vi "输入数据解析.vi"(0 "单个参数补充":dbl, 1 "从板号":dbl=1.0, 2 "主板二维码":string="BNET01", 3 "从板二维码":string="BNET01", 5 "主板引用":refnum<vi>, 7 "从板引用":refnum<vi>, 9 "主板选项":string="三级故障阀值", 11 "枚举":enum16{"主板", "从板"}(ring), 12 "快换":bool caption="快换写入") -> (4 "输出数组":dbl[][](array[numeric]), 6 "数组长度":dbl[](array[numeric]), 8 "循环次数":i32, 10 "命令":u32, 14 "名称":string[](array[string]), 15 "命令序号":u32[](array[numeric]))   [LabVIEW 2013] (continued)
                # "极柱温度过高"
                n3831 = disable-structure shown="启用" {
                  disable-tunnel: w9952 -> [w9958 _]
                  disable-tunnel: [w9954 255 ("高字节1")] -> w9950
                  frame Disabled {
                    n3832 = Unbundle By Name(w9958) -> ("极柱温度过高"=w9957:dbl)
                    n3833 = call "输入分辨率计算-EV05.vi"("1字节?"=TRUE, "数值"=w9957, "偏移量"=-40.0, "分辨率"=1.0) -> ("高字节1"=w9954:dbl)  [unwired: 1 in, 6 out]
                  }
                  frame Enabled {
                  }
                }
                n3834 = Build Array(w9950) -> (w9951:i32[])
              }
              frame 16 {
                # "SOH过低"
                n3835 = disable-structure shown="启用" {
                  disable-tunnel: [w9975 w9983] -> w9962
                  disable-tunnel: w9961 -> [w9972 _]
                  disable-tunnel: [w9964 w9983] -> w9960
                  frame Disabled {
                    n3836 = Unbundle By Name(w9972) -> ("SOH过低"=w9971:dbl)
                    n3837 = call "输入分辨率计算-EV05.vi"("1字节?"=FALSE, "数值"=w9971, "偏移量"=0.0, "分辨率"=0.1) -> ("低字节"=w9973:dbl, "高字节1"=w9974:dbl)  [unwired: 1 in, 5 out]
                    n3838 = call "二进制解析-8.6.vi"("索引"=4, "数值"=w9974) -> ("低位子数组"=w9977:i32[])  [unwired: 3 out]
                    n3839 = call "二进制解析-8.6.vi"("索引"=4, "数值"=w9973) -> ("低位子数组"=w9966:i32[], "高位子数组"=w9976:i32[])  [unwired: 2 out]
                    n3840 = call "二进制解析-8.6.vi"("索引"=4, "数值"=0) -> ("低位子数组"=w9967:i32[])  [unwired: 3 out]
                    n3841 = Insert Into Array(array=w9977, new element=w9976) -> (w9970:i32[])  [unwired: 1 in]
                    n3842 = Insert Into Array(array=w9966, new element=w9967) -> (w9965:i32[])  [unwired: 1 in]
                    n3843 = call "数值二进制转十进制-8.6.vi"("子数组"=w9970) -> ("十进制数值"=w9975:i32)  [unwired: 4 out]
                    n3844 = call "数值二进制转十进制-8.6.vi"("子数组"=w9965) -> ("十进制数值"=w9964:i32)  [unwired: 4 out]
                  }
                  frame Enabled {
                    w9983 = 255 ("高字节1")
                  }
                }
                n3845 = Build Array(w9962, w9960) -> (w9963:i32[])
              }
            }
            n3846 = Insert Into Array(array=w9768, new element=w9769) -> (w9767:dbl[])  [unwired: 1 in]
          }
          n3847 = Build Array(w9764) -> (w9763:dbl[][])
          n3848 = Build Array("三级故障阀值") -> (w9754:string[])
        }
        frame "极柱温度过高" {
          n3849 = Unbundle By Name(w9989) -> ("一级故障"=w9990:refnum<vi>)
          n3850 = property class="Clust (严格)"(reference=w9990) -> ("Value"=w9988:T4)  [unwired: 1 in, 2 out]
          n3851 = for {
            N: 17 -> [_]
            tunnel: w9988 -> [w10000]
            shift-right: [w9997] -> w9994
            shift-left: dbl[] [] -> [w9998]
            i -> [w10001]
            n3852 = case shown="13" w10001 {
              tunnel: w10000 -> [w10002 w10013 w10024 w10034 w10044 w10054 w10066 w10078 w10090 w10102 w10114 w10126 w10140 w10161 w10173 w10182 w10191]
              tunnel: [w10003 w10014 w10025 w10035 w10045 w10056 w10068 w10080 w10092 w10104 w10116 w10127 w10149 w10164 w10172 w10181 w10193] -> w9999
              frame 0, Default {
                # "总电压过高"
                n3853 = disable-structure shown="启用" {
                  disable-tunnel: [w10009 w10012] -> w10005
                  disable-tunnel: [w10008 w10012] -> w10004
                  disable-tunnel: w10002 -> [w10007 _]
                  frame Disabled {
                    n3854 = Unbundle By Name(w10007) -> ("总电压过高"=w10006:dbl)
                    n3855 = call "输入分辨率计算-EV05.vi"("1字节?"=FALSE, "数值"=w10006, "分辨率"=0.1) -> ("低字节"=w10009:dbl, "高字节1"=w10008:dbl)  [unwired: 2 in, 5 out]
                  }
                  frame Enabled {
                    w10012 = 255 ("高字节1")
                  }
                }
                n3856 = Build Array(w10004, w10005) -> (w10003:i32[])
              }
              frame 1 {
                # "总电压过低"
                n3857 = disable-structure shown="启用" {
                  disable-tunnel: [w10020 w10023] -> w10016
                  disable-tunnel: [w10019 w10023] -> w10015
                  disable-tunnel: w10013 -> [w10018 _]
                  frame Disabled {
                    n3858 = Unbundle By Name(w10018) -> ("总电压过低"=w10017:dbl)
                    n3859 = call "输入分辨率计算-EV05.vi"("1字节?"=FALSE, "数值"=w10017, "分辨率"=0.1) -> ("低字节"=w10020:dbl, "高字节1"=w10019:dbl)  [unwired: 2 in, 5 out]
                  }
                  frame Enabled {
                    w10023 = 255 ("高字节1")
                  }
                }
                n3860 = Build Array(w10015, w10016) -> (w10014:i32[])
              }
              frame 2 {
                # "温度过高"
                n3861 = disable-structure shown="启用" {
                  disable-tunnel: [w10030 255 ("高字节1")] -> w10026
                  disable-tunnel: w10024 -> [w10028 _]
                  frame Disabled {
                    n3862 = Unbundle By Name(w10028) -> ("温度过高"=w10027:dbl)
                    n3863 = call "输入分辨率计算-EV05.vi"("1字节?"=TRUE, "数值"=w10027, "偏移量"=-40.0, "分辨率"=1.0) -> ("高字节1"=w10030:dbl)  [unwired: 1 in, 6 out]
                  }
                  frame Enabled {
                  }
                }
                n3864 = Build Array(w10026) -> (w10025:i32[])
              }
              frame 3 {
                # "温度过低"
                n3865 = disable-structure shown="启用" {
                  disable-tunnel: [w10040 255 ("高字节1")] -> w10036
                  disable-tunnel: w10034 -> [w10038 _]
                  frame Disabled {
                    n3866 = Unbundle By Name(w10038) -> ("温度过低"=w10037:dbl)
                    n3867 = call "输入分辨率计算-EV05.vi"("1字节?"=TRUE, "数值"=w10037, "偏移量"=-40.0, "分辨率"=1.0) -> ("高字节1"=w10040:dbl)  [unwired: 1 in, 6 out]
                  }
                  frame Enabled {
                  }
                }
                n3868 = Build Array(w10036) -> (w10035:i32[])
              }
              frame 4 {
                # "整组温度不均衡"
                n3869 = disable-structure shown="启用" {
                  disable-tunnel: [w10050 255 ("高字节1")] -> w10046
                  disable-tunnel: w10044 -> [w10048 _]
                  frame Disabled {
                    n3870 = Unbundle By Name(w10048) -> ("整组温度不均衡"=w10047:dbl)
                    n3871 = call "输入分辨率计算-EV05.vi"("1字节?"=TRUE, "数值"=w10047, "偏移量"=0.0, "分辨率"=1.0) -> ("高字节1"=w10050:dbl)  [unwired: 1 in, 6 out]
                  }
                  frame Enabled {
                  }
                }
                n3872 = Build Array(w10046) -> (w10045:i32[])
              }
              frame 5 {
                # "单组电压不均衡"
                n3873 = disable-structure shown="启用" {
                  disable-tunnel: [w10062 w10065] -> w10057
                  disable-tunnel: [w10060 w10065] -> w10055
                  disable-tunnel: w10054 -> [w10059 _]
                  frame Disabled {
                    n3874 = Unbundle By Name(w10059) -> ("单组电压不均衡"=w10058:dbl)
                    n3875 = call "输入分辨率计算-EV05.vi"("1字节?"=FALSE, "数值"=w10058, "偏移量"=0.0, "分辨率"=0.001) -> ("低字节"=w10060:dbl, "高字节1"=w10062:dbl)  [unwired: 1 in, 5 out]
                  }
                  frame Enabled {
                    w10065 = 255 ("高字节1")
                  }
                }
                n3876 = Build Array(w10057, w10055) -> (w10056:i32[])
              }
              frame 6 {
                # "整组电压不均衡"
                n3877 = disable-structure shown="启用" {
                  disable-tunnel: [w10074 w10077] -> w10069
                  disable-tunnel: [w10072 w10077] -> w10067
                  disable-tunnel: w10066 -> [w10071 _]
                  frame Disabled {
                    n3878 = Unbundle By Name(w10071) -> ("整组电压不均衡"=w10070:dbl)
                    n3879 = call "输入分辨率计算-EV05.vi"("1字节?"=FALSE, "数值"=w10070, "偏移量"=0.0, "分辨率"=0.001) -> ("低字节"=w10072:dbl, "高字节1"=w10074:dbl)  [unwired: 1 in, 5 out]
                  }
                  frame Enabled {
                    w10077 = 255 ("高字节1")
                  }
                }
                n3880 = Build Array(w10069, w10067) -> (w10068:i32[])
              }
              frame 7 {
                # "单体电压过高"
                n3881 = disable-structure shown="启用" {
                  disable-tunnel: [w10086 w10089] -> w10081
                  disable-tunnel: [w10084 w10089] -> w10079
                  disable-tunnel: w10078 -> [w10083 _]
                  frame Disabled {
                    n3882 = Unbundle By Name(w10083) -> ("单体电压过高"=w10082:dbl)
                    n3883 = call "输入分辨率计算-EV05.vi"("1字节?"=FALSE, "数值"=w10082, "偏移量"=0.0, "分辨率"=0.001) -> ("低字节"=w10084:dbl, "高字节1"=w10086:dbl)  [unwired: 1 in, 5 out]
                  }
                  frame Enabled {
                    w10089 = 255 ("高字节1")
                  }
                }
                n3884 = Build Array(w10081, w10079) -> (w10080:i32[])
              }
              frame 8 {
                # "单体电压过低"
                n3885 = disable-structure shown="启用" {
                  disable-tunnel: [w10098 w10101] -> w10093
                  disable-tunnel: [w10096 w10101] -> w10091
                  disable-tunnel: w10090 -> [w10095 _]
                  frame Disabled {
                    n3886 = Unbundle By Name(w10095) -> ("单体电压过低"=w10094:dbl)
                    n3887 = call "输入分辨率计算-EV05.vi"("1字节?"=FALSE, "数值"=w10094, "偏移量"=0.0, "分辨率"=0.001) -> ("低字节"=w10096:dbl, "高字节1"=w10098:dbl)  [unwired: 1 in, 5 out]
                  }
                  frame Enabled {
                    w10101 = 255 ("高字节1")
                  }
                }
                n3888 = Build Array(w10093, w10091) -> (w10092:i32[])
              }
              frame 9 {
                # "充电电流过高"
                n3889 = disable-structure shown="启用" {
                  disable-tunnel: [w10110 w10113] -> w10105
                  disable-tunnel: [w10108 w10113] -> w10103
                  disable-tunnel: w10102 -> [w10107 _]
                  frame Disabled {
                    n3890 = Unbundle By Name(w10107) -> ("充电电流过高"=w10106:dbl)
                    n3891 = call "输入分辨率计算-EV05.vi"("1字节?"=FALSE, "数值"=w10106, "偏移量"=-3000.0, "分辨率"=0.1) -> ("低字节"=w10108:dbl, "高字节1"=w10110:dbl)  [unwired: 1 in, 5 out]
                  }
                  frame Enabled {
                    w10113 = 255 ("高字节1")
                  }
                }
                n3892 = Build Array(w10105, w10103) -> (w10104:i32[])
              }
              frame 10 {
                # "放电电流过高"
                n3893 = disable-structure shown="启用" {
                  disable-tunnel: [w10122 w10125] -> w10117
                  disable-tunnel: [w10120 w10125] -> w10115
                  disable-tunnel: w10114 -> [w10119 _]
                  frame Disabled {
                    n3894 = Unbundle By Name(w10119) -> ("放电电流过高"=w10118:dbl)
                    n3895 = call "输入分辨率计算-EV05.vi"("1字节?"=FALSE, "数值"=w10118, "偏移量"=-3000.0, "分辨率"=0.1) -> ("低字节"=w10120:dbl, "高字节1"=w10122:dbl)  [unwired: 1 in, 5 out]
                  }
                  frame Enabled {
                    w10125 = 255 ("高字节1")
                  }
                }
                n3896 = Build Array(w10117, w10115) -> (w10116:i32[])
              }
              frame 11 {
                # "单组温度不均衡"
                n3897 = disable-structure shown="启用" {
                  disable-tunnel: [w10132 255 ("高字节1")] -> w10128
                  disable-tunnel: w10126 -> [w10130 _]
                  frame Disabled {
                    n3898 = Unbundle By Name(w10130) -> ("单组温度不均衡"=w10129:dbl)
                    n3899 = call "输入分辨率计算-EV05.vi"("1字节?"=TRUE, "数值"=w10129, "偏移量"=0.0, "分辨率"=1.0) -> ("高字节1"=w10132:dbl)  [unwired: 1 in, 6 out]
                  }
                  frame Enabled {
                  }
                }
                n3900 = Build Array(w10128) -> (w10127:i32[])
              }
              frame 12 {
                # "SOC过高"
                n3901 = Unbundle By Name(w10140) -> ("SOC过高"=w10139:dbl)
                n3902 = call "输入分辨率计算-EV05.vi"("1字节?"=FALSE, "数值"=w10139, "偏移量"=0.0, "分辨率"=0.1) -> ("低字节"=w10141:dbl, "高字节1"=w10142:dbl)  [unwired: 1 in, 5 out]
                n3903 = call "二进制解析-8.6.vi"("索引"=4, "数值"=w10142) -> ("低位子数组"=w10145:i32[])  [unwired: 3 out]
                n3904 = call "二进制解析-8.6.vi"("索引"=4, "数值"=w10141) -> ("低位子数组"=w10137:i32[], "高位子数组"=w10144:i32[])  [unwired: 2 out]
                n3905 = Insert Into Array(array=w10145, new element=w10144) -> (w10143:i32[])  [unwired: 1 in]
                n3906 = call "数值二进制转十进制-8.6.vi"("子数组"=w10143) -> ("十进制数值"=w10138:i32)  [unwired: 4 out]
                n3907 = disable-structure shown="启用" {
                  disable-tunnel: w10138 -> [w10153 _]
                  disable-tunnel: [w10153 255 ("高字节1")] -> w10136
                  disable-tunnel: w10137 -> [w10152 _]
                  disable-tunnel: [w10152 i32[] [] ("低位子数组 29")] -> _
                  frame Disabled {
                  }
                  frame Enabled {
                  }
                }
                n3908 = Build Array(w10136, w10136) -> (w10149:i32[])
              }
              frame 13 {
                # "SOC过低"
                n3909 = Unbundle By Name(w10161) -> ("SOC过低"=w10160:dbl)
                n3910 = call "输入分辨率计算-EV05.vi"("1字节?"=FALSE, "数值"=w10160, "偏移量"=0.0, "分辨率"=0.1) -> ("低字节"=w10158:dbl, "高字节1"=w10159:dbl)  [unwired: 1 in, 5 out]
                n3911 = call "二进制解析-8.6.vi"("索引"=4, "数值"=w10159) -> ("低位子数组"=w10157:i32[])  [unwired: 3 out]
                n3912 = disable-structure shown="启用" {
                  disable-tunnel: w10158 -> [w10168 _]
                  disable-tunnel: [w10168 255 ("高字节1")] -> w10156
                  disable-tunnel: w10157 -> [w10167 _]
                  disable-tunnel: [w10167 i32[] [] ("低位子数组")] -> _
                  frame Disabled {
                    (unwired) i32[] [] ("低位子数组 4")
                  }
                  frame Enabled {
                  }
                }
                n3913 = Build Array(w10156, w10156) -> (w10164:i32[])
              }
              frame 14 {
                # "内阻过大"
                n3914 = disable-structure shown="启用" {
                  disable-tunnel: w10173 -> [w10178 _]
                  disable-tunnel: [w10174 255 ("高字节1")] -> w10171
                  frame Disabled {
                    n3915 = Unbundle By Name(w10178) -> ("内阻过大"=w10177:dbl)
                    n3916 = call "输入分辨率计算-EV05.vi"("1字节?"=TRUE, "数值"=w10177, "分辨率"=0.1) -> ("高字节1"=w10174:dbl)  [unwired: 2 in, 6 out]
                  }
                  frame Enabled {
                  }
                }
                n3917 = Build Array(w10171) -> (w10172:i32[])
              }
              frame 15 {
                # "极柱温度过高"
                n3918 = disable-structure shown="启用" {
                  disable-tunnel: w10182 -> [w10188 _]
                  disable-tunnel: [w10184 255 ("高字节1")] -> w10180
                  frame Enabled {
                    n3919 = Unbundle By Name(w10188) -> ("极柱温度过高"=w10187:dbl)
                    n3920 = call "输入分辨率计算-EV05.vi"("1字节?"=TRUE, "数值"=w10187, "偏移量"=-40.0, "分辨率"=1.0) -> ("高字节1"=w10184:dbl)  [unwired: 1 in, 6 out]
                  }
                  frame Disabled {
                  }
                }
                n3921 = Build Array(w10180) -> (w10181:dbl[])
              }
              frame 16 {
                # "SOH过低"
                n3922 = disable-structure shown="启用" {
                  disable-tunnel: [w10205 w10213] -> w10192
                  disable-tunnel: w10191 -> [w10202 _]
                  disable-tunnel: [w10194 w10213] -> w10190
                  frame Disabled {
                    n3923 = Unbundle By Name(w10202) -> ("SOH过低"=w10201:dbl)
                    n3924 = call "输入分辨率计算-EV05.vi"("1字节?"=FALSE, "数值"=w10201, "偏移量"=0.0, "分辨率"=0.1) -> ("低字节"=w10203:dbl, "高字节1"=w10204:dbl)  [unwired: 1 in, 5 out]
                    n3925 = call "二进制解析-8.6.vi"("索引"=4, "数值"=w10204) -> ("低位子数组"=w10207:i32[])  [unwired: 3 out]
                    n3926 = call "二进制解析-8.6.vi"("索引"=4, "数值"=w10203) -> ("低位子数组"=w10196:i32[], "高位子数组"=w10206:i32[])  [unwired: 2 out]
                    n3927 = call "二进制解析-8.6.vi"("索引"=4, "数值"=0) -> ("低位子数组"=w10197:i32[])  [unwired: 3 out]
                    n3928 = Insert Into Array(array=w10207, new element=w10206) -> (w10200:i32[])  [unwired: 1 in]
                    n3929 = Insert Into Array(array=w10196, new element=w10197) -> (w10195:i32[])  [unwired: 1 in]
                    n3930 = call "数值二进制转十进制-8.6.vi"("子数组"=w10200) -> ("十进制数值"=w10205:i32)  [unwired: 4 out]
                    n3931 = call "数值二进制转十进制-8.6.vi"("子数组"=w10195) -> ("十进制数值"=w10194:i32)  [unwired: 4 out]
                  }
                  frame Enabled {
                    w10213 = 255 ("高字节1")
                  }
                }
                n3932 = Build Array(w10192, w10190) -> (w10193:i32[])
              }
            }
            n3933 = Insert Into Array(array=w9998, new element=w9999) -> (w9997:dbl[])  [unwired: 1 in]
          }
          n3934 = Build Array(w9994) -> (w9993:dbl[][])
          n3935 = Build Array("一级故障阀值") -> (w9984:string[])
        }
        frame "极柱温度过高(2)" {
          n3936 = Unbundle By Name(w10219) -> ("一级故障 2"=w10220:refnum<vi>)
          n3937 = property class="Clust (严格)"(reference=w10220) -> ("Value"=w10218:T4)  [unwired: 1 in, 2 out]
          n3938 = for {
            N: 17 -> [_]
            tunnel: w10218 -> [w10230]
            shift-right: [w10227] -> w10224
            shift-left: dbl[] [] -> [w10228]
            i -> [w10231]
            n3939 = case shown="13" w10231 {
              tunnel: w10230 -> [w10232 w10243 w10254 w10264 w10274 w10284 w10296 w10308 w10320 w10332 w10344 w10356 w10370 w10391 w10403 w10412 w10421]
              tunnel: [w10233 w10244 w10255 w10265 w10275 w10286 w10298 w10310 w10322 w10334 w10346 w10357 w10379 w10394 w10402 w10411 w10423] -> w10229
              frame 0, Default {
                # "总电压过高"
                n3940 = disable-structure shown="启用" {
                  disable-tunnel: [w10239 w10242] -> w10235
                  disable-tunnel: [w10238 w10242] -> w10234
                  disable-tunnel: w10232 -> [w10237 _]
                  frame Disabled {
                    n3941 = Unbundle By Name(w10237) -> ("总电压过高"=w10236:dbl)
                    n3942 = call "输入分辨率计算-EV05.vi"("1字节?"=FALSE, "数值"=w10236, "分辨率"=0.1) -> ("低字节"=w10239:dbl, "高字节1"=w10238:dbl)  [unwired: 2 in, 5 out]
                  }
                  frame Enabled {
                    w10242 = 255 ("高字节1")
                  }
                }
                n3943 = Build Array(w10234, w10235) -> (w10233:i32[])
              }
              frame 1 {
                # "总电压过低"
                n3944 = disable-structure shown="启用" {
                  disable-tunnel: [w10250 w10253] -> w10246
                  disable-tunnel: [w10249 w10253] -> w10245
                  disable-tunnel: w10243 -> [w10248 _]
                  frame Disabled {
                    n3945 = Unbundle By Name(w10248) -> ("总电压过低"=w10247:dbl)
                    n3946 = call "输入分辨率计算-EV05.vi"("1字节?"=FALSE, "数值"=w10247, "分辨率"=0.1) -> ("低字节"=w10250:dbl, "高字节1"=w10249:dbl)  [unwired: 2 in, 5 out]
                  }
                  frame Enabled {
                    w10253 = 255 ("高字节1")
                  }
                }
                n3947 = Build Array(w10245, w10246) -> (w10244:i32[])
              }
              frame 2 {
                # "温度过高"
                n3948 = disable-structure shown="启用" {
                  disable-tunnel: [w10260 255 ("高字节1")] -> w10256
                  disable-tunnel: w10254 -> [w10258 _]
                  frame Disabled {
                    n3949 = Unbundle By Name(w10258) -> ("温度过高"=w10257:dbl)
                    n3950 = call "输入分辨率计算-EV05.vi"("1字节?"=TRUE, "数值"=w10257, "偏移量"=-40.0, "分辨率"=1.0) -> ("高字节1"=w10260:dbl)  [unwired: 1 in, 6 out]
                  }
                  frame Enabled {
                  }
                }
                n3951 = Build Array(w10256) -> (w10255:i32[])
              }
              frame 3 {
                # "温度过低"
                n3952 = disable-structure shown="启用" {
                  disable-tunnel: [w10270 255 ("高字节1")] -> w10266
                  disable-tunnel: w10264 -> [w10268 _]
                  frame Disabled {
                    n3953 = Unbundle By Name(w10268) -> ("温度过低"=w10267:dbl)
                    n3954 = call "输入分辨率计算-EV05.vi"("1字节?"=TRUE, "数值"=w10267, "偏移量"=-40.0, "分辨率"=1.0) -> ("高字节1"=w10270:dbl)  [unwired: 1 in, 6 out]
                  }
                  frame Enabled {
                  }
                }
                n3955 = Build Array(w10266) -> (w10265:i32[])
              }
              frame 4 {
                # "整组温度不均衡"
                n3956 = disable-structure shown="启用" {
                  disable-tunnel: [w10280 255 ("高字节1")] -> w10276
                  disable-tunnel: w10274 -> [w10278 _]
                  frame Disabled {
                    n3957 = Unbundle By Name(w10278) -> ("整组温度不均衡"=w10277:dbl)
                    n3958 = call "输入分辨率计算-EV05.vi"("1字节?"=TRUE, "数值"=w10277, "偏移量"=0.0, "分辨率"=1.0) -> ("高字节1"=w10280:dbl)  [unwired: 1 in, 6 out]
                  }
                  frame Enabled {
                  }
                }
                n3959 = Build Array(w10276) -> (w10275:i32[])
              }
              frame 5 {
                # "单组电压不均衡"
                n3960 = disable-structure shown="启用" {
                  disable-tunnel: [w10292 w10295] -> w10287
                  disable-tunnel: [w10290 w10295] -> w10285
                  disable-tunnel: w10284 -> [w10289 _]
                  frame Disabled {
                    n3961 = Unbundle By Name(w10289) -> ("单组电压不均衡"=w10288:dbl)
                    n3962 = call "输入分辨率计算-EV05.vi"("1字节?"=FALSE, "数值"=w10288, "偏移量"=0.0, "分辨率"=0.001) -> ("低字节"=w10290:dbl, "高字节1"=w10292:dbl)  [unwired: 1 in, 5 out]
                  }
                  frame Enabled {
                    w10295 = 255 ("高字节1")
                  }
                }
                n3963 = Build Array(w10287, w10285) -> (w10286:i32[])
              }
              frame 6 {
                # "整组电压不均衡"
                n3964 = disable-structure shown="启用" {
                  disable-tunnel: [w10304 w10307] -> w10299
                  disable-tunnel: [w10302 w10307] -> w10297
                  disable-tunnel: w10296 -> [w10301 _]
                  frame Disabled {
                    n3965 = Unbundle By Name(w10301) -> ("整组电压不均衡"=w10300:dbl)
                    n3966 = call "输入分辨率计算-EV05.vi"("1字节?"=FALSE, "数值"=w10300, "偏移量"=0.0, "分辨率"=0.001) -> ("低字节"=w10302:dbl, "高字节1"=w10304:dbl)  [unwired: 1 in, 5 out]
                  }
                  frame Enabled {
                    w10307 = 255 ("高字节1")
                  }
                }
                n3967 = Build Array(w10299, w10297) -> (w10298:i32[])
              }
              frame 7 {
                # "单体电压过高"
                n3968 = disable-structure shown="启用" {
                  disable-tunnel: [w10316 w10319] -> w10311
                  disable-tunnel: [w10314 w10319] -> w10309
                  disable-tunnel: w10308 -> [w10313 _]
                  frame Disabled {
                    n3969 = Unbundle By Name(w10313) -> ("单体电压过高"=w10312:dbl)
                    n3970 = call "输入分辨率计算-EV05.vi"("1字节?"=FALSE, "数值"=w10312, "偏移量"=0.0, "分辨率"=0.001) -> ("低字节"=w10314:dbl, "高字节1"=w10316:dbl)  [unwired: 1 in, 5 out]
                  }
                  frame Enabled {
                    w10319 = 255 ("高字节1")
                  }
                }
                n3971 = Build Array(w10311, w10309) -> (w10310:i32[])
              }
              frame 8 {
                # "单体电压过低"
                n3972 = disable-structure shown="启用" {
                  disable-tunnel: [w10328 w10331] -> w10323
                  disable-tunnel: [w10326 w10331] -> w10321
                  disable-tunnel: w10320 -> [w10325 _]
                  frame Disabled {
                    n3973 = Unbundle By Name(w10325) -> ("单体电压过低"=w10324:dbl)
                    n3974 = call "输入分辨率计算-EV05.vi"("1字节?"=FALSE, "数值"=w10324, "偏移量"=0.0, "分辨率"=0.001) -> ("低字节"=w10326:dbl, "高字节1"=w10328:dbl)  [unwired: 1 in, 5 out]
                  }
                  frame Enabled {
                    w10331 = 255 ("高字节1")
                  }
                }
                n3975 = Build Array(w10323, w10321) -> (w10322:i32[])
              }
              frame 9 {
                # "充电电流过高"
                n3976 = disable-structure shown="启用" {
                  disable-tunnel: [w10340 w10343] -> w10335
                  disable-tunnel: [w10338 w10343] -> w10333
                  disable-tunnel: w10332 -> [w10337 _]
                  frame Disabled {
                    n3977 = Unbundle By Name(w10337) -> ("充电电流过高"=w10336:dbl)
                    n3978 = call "输入分辨率计算-EV05.vi"("1字节?"=FALSE, "数值"=w10336, "偏移量"=-3000.0, "分辨率"=0.1) -> ("低字节"=w10338:dbl, "高字节1"=w10340:dbl)  [unwired: 1 in, 5 out]
                  }
                  frame Enabled {
                    w10343 = 255 ("高字节1")
                  }
                }
                n3979 = Build Array(w10335, w10333) -> (w10334:i32[])
              }
              frame 10 {
                # "放电电流过高"
                n3980 = disable-structure shown="启用" {
                  disable-tunnel: [w10352 w10355] -> w10347
                  disable-tunnel: [w10350 w10355] -> w10345
                  disable-tunnel: w10344 -> [w10349 _]
                  frame Disabled {
                    n3981 = Unbundle By Name(w10349) -> ("放电电流过高"=w10348:dbl)
                    n3982 = call "输入分辨率计算-EV05.vi"("1字节?"=FALSE, "数值"=w10348, "偏移量"=-3000.0, "分辨率"=0.1) -> ("低字节"=w10350:dbl, "高字节1"=w10352:dbl)  [unwired: 1 in, 5 out]
                  }
                  frame Enabled {
                    w10355 = 255 ("高字节1")
                  }
                }
                n3983 = Build Array(w10347, w10345) -> (w10346:i32[])
              }
              frame 11 {
                # "单组温度不均衡"
                n3984 = disable-structure shown="启用" {
                  disable-tunnel: [w10362 255 ("高字节1")] -> w10358
                  disable-tunnel: w10356 -> [w10360 _]
                  frame Disabled {
                    n3985 = Unbundle By Name(w10360) -> ("单组温度不均衡"=w10359:dbl)
                    n3986 = call "输入分辨率计算-EV05.vi"("1字节?"=TRUE, "数值"=w10359, "偏移量"=0.0, "分辨率"=1.0) -> ("高字节1"=w10362:dbl)  [unwired: 1 in, 6 out]
                  }
                  frame Enabled {
                  }
                }
                n3987 = Build Array(w10358) -> (w10357:i32[])
              }
              frame 12 {
                # "SOC过高"
                n3988 = Unbundle By Name(w10370) -> ("SOC过高"=w10369:dbl)
                n3989 = call "输入分辨率计算-EV05.vi"("1字节?"=FALSE, "数值"=w10369, "偏移量"=0.0, "分辨率"=0.1) -> ("低字节"=w10371:dbl, "高字节1"=w10372:dbl)  [unwired: 1 in, 5 out]
                n3990 = call "二进制解析-8.6.vi"("索引"=4, "数值"=w10372) -> ("低位子数组"=w10375:i32[])  [unwired: 3 out]
                n3991 = call "二进制解析-8.6.vi"("索引"=4, "数值"=w10371) -> ("低位子数组"=w10367:i32[], "高位子数组"=w10374:i32[])  [unwired: 2 out]
                n3992 = Insert Into Array(array=w10375, new element=w10374) -> (w10373:i32[])  [unwired: 1 in]
                n3993 = call "数值二进制转十进制-8.6.vi"("子数组"=w10373) -> ("十进制数值"=w10368:i32)  [unwired: 4 out]
                n3994 = disable-structure shown="启用" {
                  disable-tunnel: w10368 -> [w10383 _]
                  disable-tunnel: [w10383 255 ("高字节1")] -> w10366
                  disable-tunnel: w10367 -> [w10382 _]
                  disable-tunnel: [w10382 i32[] [] ("低位子数组 29")] -> _
                  frame Disabled {
                  }
                  frame Enabled {
                  }
                }
                n3995 = Build Array(w10366, w10366) -> (w10379:i32[])
              }
              frame 13 {
                # "SOC过低"
                n3996 = Unbundle By Name(w10391) -> ("SOC过低"=w10390:dbl)
                n3997 = call "输入分辨率计算-EV05.vi"("1字节?"=FALSE, "数值"=w10390, "偏移量"=0.0, "分辨率"=0.1) -> ("低字节"=w10388:dbl, "高字节1"=w10389:dbl)  [unwired: 1 in, 5 out]
                n3998 = call "二进制解析-8.6.vi"("索引"=4, "数值"=w10389) -> ("低位子数组"=w10387:i32[])  [unwired: 3 out]
                n3999 = disable-structure shown="启用" {
                  disable-tunnel: w10388 -> [w10398 _]
                  disable-tunnel: [w10398 255 ("高字节1")] -> w10386
                  disable-tunnel: w10387 -> [w10397 _]
                  disable-tunnel: [w10397 i32[] [] ("低位子数组")] -> _
                  frame Disabled {
                    (unwired) i32[] [] ("低位子数组 4")
                  }
                  frame Enabled {
                  }
                }
                n4000 = Build Array(w10386, w10386) -> (w10394:i32[])
              }
              frame 14 {
                # "内阻过大"
                n4001 = disable-structure shown="启用" {
                  disable-tunnel: w10403 -> [w10408 _]
                  disable-tunnel: [w10404 255 ("高字节1")] -> w10401
                  frame Disabled {
                    n4002 = Unbundle By Name(w10408) -> ("内阻过大"=w10407:dbl)
                    n4003 = call "输入分辨率计算-EV05.vi"("1字节?"=TRUE, "数值"=w10407, "分辨率"=0.1) -> ("高字节1"=w10404:dbl)  [unwired: 2 in, 6 out]
                  }
                  frame Enabled {
                  }
                }
                n4004 = Build Array(w10401) -> (w10402:i32[])
              }
              frame 15 {
                # "极柱温度过高"
                n4005 = disable-structure shown="启用" {
                  disable-tunnel: w10412 -> [w10418 _]
                  disable-tunnel: [w10414 255 ("高字节1")] -> w10410
                  frame Enabled {
                    n4006 = Unbundle By Name(w10418) -> ("极柱温度过高"=w10417:dbl)
                    n4007 = call "输入分辨率计算-EV05.vi"("1字节?"=TRUE, "数值"=w10417, "偏移量"=-40.0, "分辨率"=1.0) -> ("高字节1"=w10414:dbl)  [unwired: 1 in, 6 out]
                  }
                  frame Disabled {
                  }
                }
                n4008 = Build Array(w10410) -> (w10411:dbl[])
              }
              frame 16 {
                # "SOH过低"
                n4009 = disable-structure shown="启用" {
                  disable-tunnel: [w10435 w10443] -> w10422
                  disable-tunnel: w10421 -> [w10432 _]
                  disable-tunnel: [w10424 w10443] -> w10420
                  frame Disabled {
                    n4010 = Unbundle By Name(w10432) -> ("SOH过低"=w10431:dbl)
                    n4011 = call "输入分辨率计算-EV05.vi"("1字节?"=FALSE, "数值"=w10431, "偏移量"=0.0, "分辨率"=0.1) -> ("低字节"=w10433:dbl, "高字节1"=w10434:dbl)  [unwired: 1 in, 5 out]
                    n4012 = call "二进制解析-8.6.vi"("索引"=4, "数值"=w10434) -> ("低位子数组"=w10437:i32[])  [unwired: 3 out]
                    n4013 = call "二进制解析-8.6.vi"("索引"=4, "数值"=w10433) -> ("低位子数组"=w10426:i32[], "高位子数组"=w10436:i32[])  [unwired: 2 out]
                    n4014 = call "二进制解析-8.6.vi"("索引"=4, "数值"=0) -> ("低位子数组"=w10427:i32[])  [unwired: 3 out]
                    n4015 = Insert Into Array(array=w10437, new element=w10436) -> (w10430:i32[])  [unwired: 1 in]
                    n4016 = Insert Into Array(array=w10426, new element=w10427) -> (w10425:i32[])  [unwired: 1 in]
                    n4017 = call "数值二进制转十进制-8.6.vi"("子数组"=w10430) -> ("十进制数值"=w10435:i32)  [unwired: 4 out]
                    n4018 = call "数值二进制转十进制-8.6.vi"("子数组"=w10425) -> ("十进制数值"=w10424:i32)  [unwired: 4 out]
                  }
                  frame Enabled {
                    w10443 = 255 ("高字节1")
                  }
                }
                n4019 = Build Array(w10422, w10420) -> (w10423:i32[])
              }
            }
            n4020 = Insert Into Array(array=w10228, new element=w10229) -> (w10227:dbl[])  [unwired: 1 in]
          }
          n4021 = Build Array(w10224) -> (w10223:dbl[][])
          n4022 = Build Array("二级故障阀值") -> (w10214:string[])
        }
        frame "极柱温度过高(3)" {
          n4023 = Unbundle By Name(w10449) -> ("一级故障 3"=w10450:refnum<vi>)
          n4024 = property class="Clust (严格)"(reference=w10450) -> ("Value"=w10448:T4)  [unwired: 1 in, 2 out]
          n4025 = for {
            N: 17 -> [_]
            tunnel: w10448 -> [w10460]
            shift-right: [w10457] -> w10454
            shift-left: dbl[] [] -> [w10458]
            i -> [w10461]
            n4026 = case shown="13" w10461 {
              tunnel: w10460 -> [w10462 w10473 w10484 w10494 w10504 w10514 w10526 w10538 w10550 w10562 w10574 w10586 w10600 w10621 w10633 w10642 w10651]
              tunnel: [w10463 w10474 w10485 w10495 w10505 w10516 w10528 w10540 w10552 w10564 w10576 w10587 w10609 w10624 w10632 w10641 w10653] -> w10459
              frame 0, Default {
                # "总电压过高"
                n4027 = disable-structure shown="启用" {
                  disable-tunnel: [w10469 w10472] -> w10465
                  disable-tunnel: [w10468 w10472] -> w10464
                  disable-tunnel: w10462 -> [w10467 _]
                  frame Disabled {
                    n4028 = Unbundle By Name(w10467) -> ("总电压过高"=w10466:dbl)
                    n4029 = call "输入分辨率计算-EV05.vi"("1字节?"=FALSE, "数值"=w10466, "分辨率"=0.1) -> ("低字节"=w10469:dbl, "高字节1"=w10468:dbl)  [unwired: 2 in, 5 out]
                  }
                  frame Enabled {
                    w10472 = 255 ("高字节1")
                  }
                }
                n4030 = Build Array(w10464, w10465) -> (w10463:i32[])
              }
              frame 1 {
                # "总电压过低"
                n4031 = disable-structure shown="启用" {
                  disable-tunnel: [w10480 w10483] -> w10476
                  disable-tunnel: [w10479 w10483] -> w10475
                  disable-tunnel: w10473 -> [w10478 _]
                  frame Disabled {
                    n4032 = Unbundle By Name(w10478) -> ("总电压过低"=w10477:dbl)
                    n4033 = call "输入分辨率计算-EV05.vi"("1字节?"=FALSE, "数值"=w10477, "分辨率"=0.1) -> ("低字节"=w10480:dbl, "高字节1"=w10479:dbl)  [unwired: 2 in, 5 out]
                  }
                  frame Enabled {
                    w10483 = 255 ("高字节1")
                  }
                }
                n4034 = Build Array(w10475, w10476) -> (w10474:i32[])
              }
              frame 2 {
                # "温度过高"
                n4035 = disable-structure shown="启用" {
                  disable-tunnel: [w10490 255 ("高字节1")] -> w10486
                  disable-tunnel: w10484 -> [w10488 _]
                  frame Disabled {
                    n4036 = Unbundle By Name(w10488) -> ("温度过高"=w10487:dbl)
                    n4037 = call "输入分辨率计算-EV05.vi"("1字节?"=TRUE, "数值"=w10487, "偏移量"=-40.0, "分辨率"=1.0) -> ("高字节1"=w10490:dbl)  [unwired: 1 in, 6 out]
                  }
                  frame Enabled {
                  }
                }
                n4038 = Build Array(w10486) -> (w10485:i32[])
              }
              frame 3 {
                # "温度过低"
                n4039 = disable-structure shown="启用" {
                  disable-tunnel: [w10500 255 ("高字节1")] -> w10496
                  disable-tunnel: w10494 -> [w10498 _]
                  frame Disabled {
                    n4040 = Unbundle By Name(w10498) -> ("温度过低"=w10497:dbl)
                    n4041 = call "输入分辨率计算-EV05.vi"("1字节?"=TRUE, "数值"=w10497, "偏移量"=-40.0, "分辨率"=1.0) -> ("高字节1"=w10500:dbl)  [unwired: 1 in, 6 out]
                  }
                  frame Enabled {
                  }
                }
                n4042 = Build Array(w10496) -> (w10495:i32[])
              }
              frame 4 {
                # "整组温度不均衡"
                n4043 = disable-structure shown="启用" {
                  disable-tunnel: [w10510 255 ("高字节1")] -> w10506
                  disable-tunnel: w10504 -> [w10508 _]
                  frame Disabled {
                    n4044 = Unbundle By Name(w10508) -> ("整组温度不均衡"=w10507:dbl)
                    n4045 = call "输入分辨率计算-EV05.vi"("1字节?"=TRUE, "数值"=w10507, "偏移量"=0.0, "分辨率"=1.0) -> ("高字节1"=w10510:dbl)  [unwired: 1 in, 6 out]
                  }
                  frame Enabled {
                  }
                }
                n4046 = Build Array(w10506) -> (w10505:i32[])
              }
              frame 5 {
                # "单组电压不均衡"
                n4047 = disable-structure shown="启用" {
                  disable-tunnel: [w10522 w10525] -> w10517
                  disable-tunnel: [w10520 w10525] -> w10515
                  disable-tunnel: w10514 -> [w10519 _]
                  frame Disabled {
                    n4048 = Unbundle By Name(w10519) -> ("单组电压不均衡"=w10518:dbl)
                    n4049 = call "输入分辨率计算-EV05.vi"("1字节?"=FALSE, "数值"=w10518, "偏移量"=0.0, "分辨率"=0.001) -> ("低字节"=w10520:dbl, "高字节1"=w10522:dbl)  [unwired: 1 in, 5 out]
                  }
                  frame Enabled {
                    w10525 = 255 ("高字节1")
                  }
                }
                n4050 = Build Array(w10517, w10515) -> (w10516:i32[])
              }
              frame 6 {
                # "整组电压不均衡"
                n4051 = disable-structure shown="启用" {
                  disable-tunnel: [w10534 w10537] -> w10529
                  disable-tunnel: [w10532 w10537] -> w10527
                  disable-tunnel: w10526 -> [w10531 _]
                  frame Disabled {
                    n4052 = Unbundle By Name(w10531) -> ("整组电压不均衡"=w10530:dbl)
                    n4053 = call "输入分辨率计算-EV05.vi"("1字节?"=FALSE, "数值"=w10530, "偏移量"=0.0, "分辨率"=0.001) -> ("低字节"=w10532:dbl, "高字节1"=w10534:dbl)  [unwired: 1 in, 5 out]
                  }
                  frame Enabled {
                    w10537 = 255 ("高字节1")
                  }
                }
                n4054 = Build Array(w10529, w10527) -> (w10528:i32[])
              }
              frame 7 {
                # "单体电压过高"
                n4055 = disable-structure shown="启用" {
                  disable-tunnel: [w10546 w10549] -> w10541
                  disable-tunnel: [w10544 w10549] -> w10539
                  disable-tunnel: w10538 -> [w10543 _]
                  frame Disabled {
                    n4056 = Unbundle By Name(w10543) -> ("单体电压过高"=w10542:dbl)
                    n4057 = call "输入分辨率计算-EV05.vi"("1字节?"=FALSE, "数值"=w10542, "偏移量"=0.0, "分辨率"=0.001) -> ("低字节"=w10544:dbl, "高字节1"=w10546:dbl)  [unwired: 1 in, 5 out]
                  }
                  frame Enabled {
                    w10549 = 255 ("高字节1")
                  }
                }
                n4058 = Build Array(w10541, w10539) -> (w10540:i32[])
              }
              frame 8 {
                # "单体电压过低"
                n4059 = disable-structure shown="启用" {
                  disable-tunnel: [w10558 w10561] -> w10553
                  disable-tunnel: [w10556 w10561] -> w10551
                  disable-tunnel: w10550 -> [w10555 _]
                  frame Disabled {
                    n4060 = Unbundle By Name(w10555) -> ("单体电压过低"=w10554:dbl)
                    n4061 = call "输入分辨率计算-EV05.vi"("1字节?"=FALSE, "数值"=w10554, "偏移量"=0.0, "分辨率"=0.001) -> ("低字节"=w10556:dbl, "高字节1"=w10558:dbl)  [unwired: 1 in, 5 out]
                  }
                  frame Enabled {
                    w10561 = 255 ("高字节1")
                  }
                }
                n4062 = Build Array(w10553, w10551) -> (w10552:i32[])
              }
              frame 9 {
                # "充电电流过高"
                n4063 = disable-structure shown="启用" {
                  disable-tunnel: [w10570 w10573] -> w10565
                  disable-tunnel: [w10568 w10573] -> w10563
                  disable-tunnel: w10562 -> [w10567 _]
                  frame Disabled {
                    n4064 = Unbundle By Name(w10567) -> ("充电电流过高"=w10566:dbl)
                    n4065 = call "输入分辨率计算-EV05.vi"("1字节?"=FALSE, "数值"=w10566, "偏移量"=-3000.0, "分辨率"=0.1) -> ("低字节"=w10568:dbl, "高字节1"=w10570:dbl)  [unwired: 1 in, 5 out]
                  }
                  frame Enabled {
                    w10573 = 255 ("高字节1")
                  }
                }
                n4066 = Build Array(w10565, w10563) -> (w10564:i32[])
              }
              frame 10 {
                # "放电电流过高"
                n4067 = disable-structure shown="启用" {
                  disable-tunnel: [w10582 w10585] -> w10577
                  disable-tunnel: [w10580 w10585] -> w10575
                  disable-tunnel: w10574 -> [w10579 _]
                  frame Disabled {
                    n4068 = Unbundle By Name(w10579) -> ("放电电流过高"=w10578:dbl)
                    n4069 = call "输入分辨率计算-EV05.vi"("1字节?"=FALSE, "数值"=w10578, "偏移量"=-3000.0, "分辨率"=0.1) -> ("低字节"=w10580:dbl, "高字节1"=w10582:dbl)  [unwired: 1 in, 5 out]
                  }
                  frame Enabled {
                    w10585 = 255 ("高字节1")
                  }
                }
                n4070 = Build Array(w10577, w10575) -> (w10576:i32[])
              }
              frame 11 {
                # "单组温度不均衡"
                n4071 = disable-structure shown="启用" {
                  disable-tunnel: [w10592 255 ("高字节1")] -> w10588
                  disable-tunnel: w10586 -> [w10590 _]
                  frame Disabled {
                    n4072 = Unbundle By Name(w10590) -> ("单组温度不均衡"=w10589:dbl)
                    n4073 = call "输入分辨率计算-EV05.vi"("1字节?"=TRUE, "数值"=w10589, "偏移量"=0.0, "分辨率"=1.0) -> ("高字节1"=w10592:dbl)  [unwired: 1 in, 6 out]
                  }
                  frame Enabled {
                  }
                }
                n4074 = Build Array(w10588) -> (w10587:i32[])
              }
              frame 12 {
                # "SOC过高"
                n4075 = Unbundle By Name(w10600) -> ("SOC过高"=w10599:dbl)
                n4076 = call "输入分辨率计算-EV05.vi"("1字节?"=FALSE, "数值"=w10599, "偏移量"=0.0, "分辨率"=0.1) -> ("低字节"=w10601:dbl, "高字节1"=w10602:dbl)  [unwired: 1 in, 5 out]
                n4077 = call "二进制解析-8.6.vi"("索引"=4, "数值"=w10602) -> ("低位子数组"=w10605:i32[])  [unwired: 3 out]
                n4078 = call "二进制解析-8.6.vi"("索引"=4, "数值"=w10601) -> ("低位子数组"=w10597:i32[], "高位子数组"=w10604:i32[])  [unwired: 2 out]
                n4079 = Insert Into Array(array=w10605, new element=w10604) -> (w10603:i32[])  [unwired: 1 in]
                n4080 = call "数值二进制转十进制-8.6.vi"("子数组"=w10603) -> ("十进制数值"=w10598:i32)  [unwired: 4 out]
                n4081 = disable-structure shown="启用" {
                  disable-tunnel: w10598 -> [w10613 _]
                  disable-tunnel: [w10613 255 ("高字节1")] -> w10596
                  disable-tunnel: w10597 -> [w10612 _]
                  disable-tunnel: [w10612 i32[] [] ("低位子数组 29")] -> _
                  frame Disabled {
                  }
                  frame Enabled {
                  }
                }
                n4082 = Build Array(w10596, w10596) -> (w10609:i32[])
              }
              frame 13 {
                # "SOC过低"
                n4083 = Unbundle By Name(w10621) -> ("SOC过低"=w10620:dbl)
                n4084 = call "输入分辨率计算-EV05.vi"("1字节?"=FALSE, "数值"=w10620, "偏移量"=0.0, "分辨率"=0.1) -> ("低字节"=w10618:dbl, "高字节1"=w10619:dbl)  [unwired: 1 in, 5 out]
                n4085 = call "二进制解析-8.6.vi"("索引"=4, "数值"=w10619) -> ("低位子数组"=w10617:i32[])  [unwired: 3 out]
                n4086 = disable-structure shown="启用" {
                  disable-tunnel: w10618 -> [w10628 _]
                  disable-tunnel: [w10628 255 ("高字节1")] -> w10616
                  disable-tunnel: w10617 -> [w10627 _]
                  disable-tunnel: [w10627 i32[] [] ("低位子数组")] -> _
                  frame Disabled {
                    (unwired) i32[] [] ("低位子数组 4")
                  }
                  frame Enabled {
                  }
                }
                n4087 = Build Array(w10616, w10616) -> (w10624:i32[])
              }
              frame 14 {
                # "内阻过大"
                n4088 = disable-structure shown="启用" {
                  disable-tunnel: w10633 -> [w10638 _]
                  disable-tunnel: [w10634 255 ("高字节1")] -> w10631
                  frame Disabled {
                    n4089 = Unbundle By Name(w10638) -> ("内阻过大"=w10637:dbl)
                    n4090 = call "输入分辨率计算-EV05.vi"("1字节?"=TRUE, "数值"=w10637, "分辨率"=0.1) -> ("高字节1"=w10634:dbl)  [unwired: 2 in, 6 out]
                  }
                  frame Enabled {
                  }
                }
                n4091 = Build Array(w10631) -> (w10632:i32[])
              }
              frame 15 {
                # "极柱温度过高"
                n4092 = disable-structure shown="启用" {
                  disable-tunnel: w10642 -> [w10648 _]
                  disable-tunnel: [w10644 255 ("高字节1")] -> w10640
                  frame Enabled {
                    n4093 = Unbundle By Name(w10648) -> ("极柱温度过高"=w10647:dbl)
                    n4094 = call "输入分辨率计算-EV05.vi"("1字节?"=TRUE, "数值"=w10647, "偏移量"=-40.0, "分辨率"=1.0) -> ("高字节1"=w10644:dbl)  [unwired: 1 in, 6 out]
                  }
                  frame Disabled {
                  }
                }
                n4095 = Build Array(w10640) -> (w10641:dbl[])
              }
              frame 16 {
                # "SOH过低"
                n4096 = disable-structure shown="启用" {
                  disable-tunnel: [w10665 w10673] -> w10652
                  disable-tunnel: w10651 -> [w10662 _]
                  disable-tunnel: [w10654 w10673] -> w10650
                  frame Disabled {
                    n4097 = Unbundle By Name(w10662) -> ("SOH过低"=w10661:dbl)
                    n4098 = call "输入分辨率计算-EV05.vi"("1字节?"=FALSE, "数值"=w10661, "偏移量"=0.0, "分辨率"=0.1) -> ("低字节"=w10663:dbl, "高字节1"=w10664:dbl)  [unwired: 1 in, 5 out]
                    n4099 = call "二进制解析-8.6.vi"("索引"=4, "数值"=w10664) -> ("低位子数组"=w10667:i32[])  [unwired: 3 out]
                    n4100 = call "二进制解析-8.6.vi"("索引"=4, "数值"=w10663) -> ("低位子数组"=w10656:i32[], "高位子数组"=w10666:i32[])  [unwired: 2 out]
                    n4101 = call "二进制解析-8.6.vi"("索引"=4, "数值"=0) -> ("低位子数组"=w10657:i32[])  [unwired: 3 out]
                    n4102 = Insert Into Array(array=w10667, new element=w10666) -> (w10660:i32[])  [unwired: 1 in]
                    n4103 = Insert Into Array(array=w10656, new element=w10657) -> (w10655:i32[])  [unwired: 1 in]
                    n4104 = call "数值二进制转十进制-8.6.vi"("子数组"=w10660) -> ("十进制数值"=w10665:i32)  [unwired: 4 out]
                    n4105 = call "数值二进制转十进制-8.6.vi"("子数组"=w10655) -> ("十进制数值"=w10654:i32)  [unwired: 4 out]
                  }
                  frame Enabled {
                    w10673 = 255 ("高字节1")
                  }
                }
                n4106 = Build Array(w10652, w10650) -> (w10653:i32[])
              }
            }
            n4107 = Insert Into Array(array=w10458, new element=w10459) -> (w10457:dbl[])  [unwired: 1 in]
          }
          n4108 = Build Array(w10454) -> (w10453:dbl[][])
          n4109 = Build Array("三级故障阀值") -> (w10444:string[])
        }
        frame "SOH过低" {
          n4110 = Unbundle By Name(w10679) -> ("一级故障"=w10680:refnum<vi>)
          n4111 = property class="Clust (严格)"(reference=w10680) -> ("Value"=w10678:T4)  [unwired: 1 in, 2 out]
          n4112 = for {
            N: 17 -> [_]
            tunnel: w10678 -> [w10690]
            shift-right: [w10687] -> w10684
            shift-left: dbl[] [] -> [w10688]
            i -> [w10691]
            n4113 = case shown="13" w10691 {
              tunnel: w10690 -> [w10692 w10703 w10714 w10724 w10734 w10744 w10756 w10768 w10780 w10792 w10804 w10816 w10830 w10851 w10864 w10873 w10882]
              tunnel: [w10693 w10704 w10715 w10725 w10735 w10746 w10758 w10770 w10782 w10794 w10806 w10817 w10839 w10854 w10863 w10872 w10884] -> w10689
              frame 0, Default {
                # "总电压过高"
                n4114 = disable-structure shown="启用" {
                  disable-tunnel: [w10699 w10702] -> w10695
                  disable-tunnel: [w10698 w10702] -> w10694
                  disable-tunnel: w10692 -> [w10697 _]
                  frame Disabled {
                    n4115 = Unbundle By Name(w10697) -> ("总电压过高"=w10696:dbl)
                    n4116 = call "输入分辨率计算-EV05.vi"("1字节?"=FALSE, "数值"=w10696, "分辨率"=0.1) -> ("低字节"=w10699:dbl, "高字节1"=w10698:dbl)  [unwired: 2 in, 5 out]
                  }
                  frame Enabled {
                    w10702 = 255 ("高字节1")
                  }
                }
                n4117 = Build Array(w10694, w10695) -> (w10693:i32[])
              }
              frame 1 {
                # "总电压过低"
                n4118 = disable-structure shown="启用" {
                  disable-tunnel: [w10710 w10713] -> w10706
                  disable-tunnel: [w10709 w10713] -> w10705
                  disable-tunnel: w10703 -> [w10708 _]
                  frame Disabled {
                    n4119 = Unbundle By Name(w10708) -> ("总电压过低"=w10707:dbl)
                    n4120 = call "输入分辨率计算-EV05.vi"("1字节?"=FALSE, "数值"=w10707, "分辨率"=0.1) -> ("低字节"=w10710:dbl, "高字节1"=w10709:dbl)  [unwired: 2 in, 5 out]
                  }
                  frame Enabled {
                    w10713 = 255 ("高字节1")
                  }
                }
                n4121 = Build Array(w10705, w10706) -> (w10704:i32[])
              }
              frame 2 {
                # "温度过高"
                n4122 = disable-structure shown="启用" {
                  disable-tunnel: [w10720 255 ("高字节1")] -> w10716
                  disable-tunnel: w10714 -> [w10718 _]
                  frame Disabled {
                    n4123 = Unbundle By Name(w10718) -> ("温度过高"=w10717:dbl)
                    n4124 = call "输入分辨率计算-EV05.vi"("1字节?"=TRUE, "数值"=w10717, "偏移量"=-40.0, "分辨率"=1.0) -> ("高字节1"=w10720:dbl)  [unwired: 1 in, 6 out]
                  }
                  frame Enabled {
                  }
                }
                n4125 = Build Array(w10716) -> (w10715:i32[])
              }
              frame 3 {
                # "温度过低"
                n4126 = disable-structure shown="启用" {
                  disable-tunnel: [w10730 255 ("高字节1")] -> w10726
                  disable-tunnel: w10724 -> [w10728 _]
                  frame Disabled {
                    n4127 = Unbundle By Name(w10728) -> ("温度过低"=w10727:dbl)
                    n4128 = call "输入分辨率计算-EV05.vi"("1字节?"=TRUE, "数值"=w10727, "偏移量"=-40.0, "分辨率"=1.0) -> ("高字节1"=w10730:dbl)  [unwired: 1 in, 6 out]
                  }
                  frame Enabled {
                  }
                }
                n4129 = Build Array(w10726) -> (w10725:i32[])
              }
              frame 4 {
                # "整组温度不均衡"
                n4130 = disable-structure shown="启用" {
                  disable-tunnel: [w10740 255 ("高字节1")] -> w10736
                  disable-tunnel: w10734 -> [w10738 _]
                  frame Disabled {
                    n4131 = Unbundle By Name(w10738) -> ("整组温度不均衡"=w10737:dbl)
                    n4132 = call "输入分辨率计算-EV05.vi"("1字节?"=TRUE, "数值"=w10737, "偏移量"=0.0, "分辨率"=1.0) -> ("高字节1"=w10740:dbl)  [unwired: 1 in, 6 out]
                  }
                  frame Enabled {
                  }
                }
                n4133 = Build Array(w10736) -> (w10735:i32[])
              }
              frame 5 {
                # "单组电压不均衡"
                n4134 = disable-structure shown="启用" {
                  disable-tunnel: [w10752 w10755] -> w10747
                  disable-tunnel: [w10750 w10755] -> w10745
                  disable-tunnel: w10744 -> [w10749 _]
                  frame Disabled {
                    n4135 = Unbundle By Name(w10749) -> ("单组电压不均衡"=w10748:dbl)
                    n4136 = call "输入分辨率计算-EV05.vi"("1字节?"=FALSE, "数值"=w10748, "偏移量"=0.0, "分辨率"=0.001) -> ("低字节"=w10750:dbl, "高字节1"=w10752:dbl)  [unwired: 1 in, 5 out]
                  }
                  frame Enabled {
                    w10755 = 255 ("高字节1")
                  }
                }
                n4137 = Build Array(w10747, w10745) -> (w10746:i32[])
              }
              frame 6 {
                # "整组电压不均衡"
                n4138 = disable-structure shown="启用" {
                  disable-tunnel: [w10764 w10767] -> w10759
                  disable-tunnel: [w10762 w10767] -> w10757
                  disable-tunnel: w10756 -> [w10761 _]
                  frame Disabled {
                    n4139 = Unbundle By Name(w10761) -> ("整组电压不均衡"=w10760:dbl)
                    n4140 = call "输入分辨率计算-EV05.vi"("1字节?"=FALSE, "数值"=w10760, "偏移量"=0.0, "分辨率"=0.001) -> ("低字节"=w10762:dbl, "高字节1"=w10764:dbl)  [unwired: 1 in, 5 out]
                  }
